vi "ExpectedSumAndRxSum (SubVI).vi"(10 "Header in":string, 11 "Numeric Control":u16) -> (3 "Equal?":bool)   [LabVIEW 2017]
panel:
  out "RxSum":u16 format="%.0x"
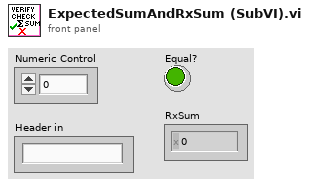
[diagram p1: front panel]
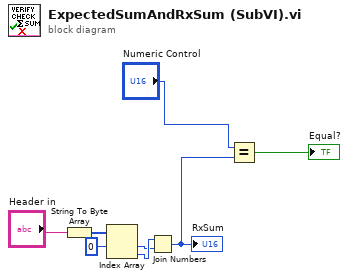
[diagram p0: block diagram]
diagram:
  n1 = String To Byte Array(string="Header in") -> (unsigned byte array=w2:u8[])
  n2 = Index Array(array=w2, index #1=0 ("index")) -> (element #1=w4:u8, element #2=w5:u8)  [unwired: 1 in]
  n3 = Join Numbers(hi=w5, lo=w4) -> ((hi.lo)=w7:u16)
  "RxSum" <- w7
  n4 = Equal?(x="Numeric Control", y=w7) -> (x = y?=→"Equal?":bool)
